vi "LVPortRealToMatlabScriptNodeSetValue.vi"(10 "Container Type":T1, 11 "Value":variant) -> (2 "1D Array":dbl[](array[numeric]), 3 "Size(s)":u32[](array[numeric]))   [LabVIEW 2017]
uses:
  Common/ObjectMap/LVPortObjectMapContainerTypeEnum.ctl
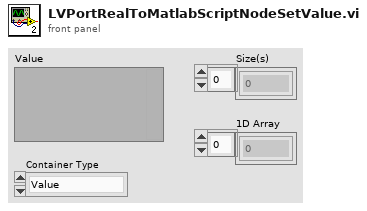
[diagram p1: front panel]
types:
  T1 = typedef "LVPortObjectMapContainerTypeEnum.ctl" = enum16{"Value", "Array", "Waveform"}
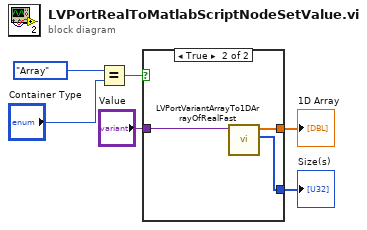
[diagram p0: block diagram]
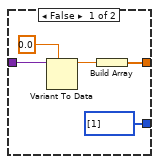
[diagram p2: hidden frame]
diagram:
  n1 = Equal?(x=LVPortObjectMapContainerTypeEnum."Array" ("Container Type"), y="Container Type") -> (x = y?=w5:bool)
  n2 = case shown="True" w5 {
    tunnel: [w9 w14] -> w2
    tunnel: [u32[] [1] ("Size(s)") w13] -> w3
    tunnel: "Value" -> [w7 w12]
    frame False {
      n3 = Variant To Data(type=0.0, Variant=w7) -> (data=w10:dbl)  [unwired: 1 in, 1 out]
      n4 = Build Array(w10) -> (w9:dbl[])
    }
    frame True {
      n5 = call "LVPortVariantArrayTo1DArrayOfRealFast.vi"("Variant Real Array"=w12) -> ("Size(s)"=w13:u32[], "1D Array"=w14:dbl[])  [unwired: 8 in, 1 out]
    }
  }
  "Size(s)" <- w3
  "1D Array" <- w2
